vi "Utility Delay ON.vi"(10 "Delay Time":dbl, 11 "Input":bool) -> (3 "Output":bool)   [LabVIEW 2017]
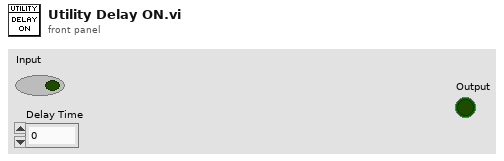
[diagram p1: front panel]
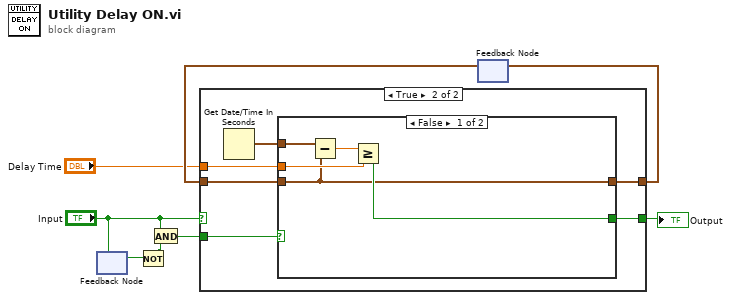
[diagram p0: block diagram]
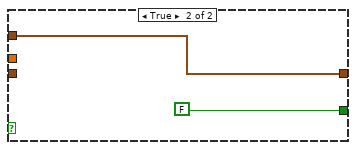
[diagram p3: hidden frame]
diagram:
  n1 = feedback #1() -> (w7:bool)  [unwired: 1 in]
  n2 = feedback-in #1("Input") -> ()
  n3 = Not(x=w7) -> (.not. x?=w8:bool)
  n4 = And(x="Input", y=w8) -> (x .and. y?=w5:bool)
  n5 = feedback #2() -> (w3:timestamp)  [unwired: 1 in]
  n6 = case shown="True" "Input" {
    selector: "Input" -> [w10 _]
    tunnel: w5 -> [_ w14]
    tunnel: [w9 w16] -> w4
    tunnel: w3 -> [w9 w15]
    tunnel: "Delay Time" -> [_ w13]
    tunnel: [w10 w12] -> w1
    frame False {
    }
    frame True {
      n7 = Get Date/Time In Seconds() -> (seconds since 1Jan1904=w11:timestamp)
      n8 = case shown="False" w14 {
        tunnel: w11 -> [w21 w23]
        tunnel: [w17 w23] -> w16
        tunnel: w15 -> [w17 _]
        tunnel: w13 -> [w19 _]
        tunnel: [w18 FALSE] -> w12
        frame False {
          n9 = Subtract(x=w21, y=w17) -> (x-y=w20:dbl)
          n10 = Greater Or Equal?(x=w20, y=w19) -> (x >= y?=w18:bool)
        }
        frame True {
        }
      }
    }
  }
  "Output" <- w1
  n11 = feedback-in #2(w4) -> ()
